vi "TiePie.Gen.Start.vi"(8 "error in (no error)":errorcluster, 11 "GenHandle":T1) -> (0 "error out":errorcluster, 3 "GenHandle out":T1)   [LabVIEW 2013, in "LVTiePie.lvlib"]
uses:
  LVTiePie.lvlib
  TiePie.Gen.handle.ctl
  bin/libtiepie.dll
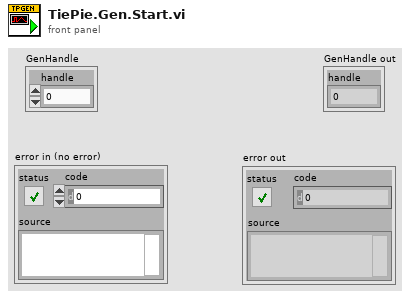
[diagram p1: front panel]
types:
  T1 = typedef "TiePie.Gen.handle.ctl" = cluster{"handle":u32}
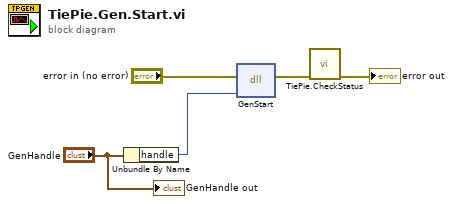
[diagram p0: block diagram]
diagram:
  n1 = Unbundle By Name("GenHandle") -> ("handle"=w4:u32)
  n2 = dll-call lib="D:/Documents and Settings/XP/Moje dokumenty/acas/trunk/support_projects/ACAS_QY/sources/drivers/LVTiePie/bin/libtiepie.dll" fn="GenStart"(error in="error in (no error)", "handle"=w4) -> (error out=w2:errorcluster)  [unwired: 4 in, 1 out]
  n3 = call "TiePie.CheckStatus.vi"("error in (no error)"=w2) -> ("error out"=→"error out":errorcluster)  [unwired: 10 in]
  "GenHandle out" <- "GenHandle"
